vi "PCO_GetHWIOSignal.vi"(8 "error in (no error)":errorcluster {"code" format="%x"}, 10 "wSignalNum":u16, 11 "ph":u64) -> (0 "error out":errorcluster {"code" format="%x"}, 1 "strSignal":T1, 2 "ErrorMessage":i32 format="%x", 3 "ph out":u64)   [LabVIEW 2019, in "SDK.lvlib" / "TimingControl.lvlib"]
doc: "<b>Description:</b>\nThis function returns the current settings of a distinct hardware input/output (IO) signal line. To select the setting for a signal line use PCO_SetHWIOSignal.\n\n<b>Supported camera type:</b>\npco.edge, pco.dimax\n\n<b>Descriptor dependency:</b>\ndwGeneralCapsDESC1: HW_IO_SIGNAL_DESCRIPTOR"
uses:
  TimingControl.lvlib
  Structures/Structures.lvlib
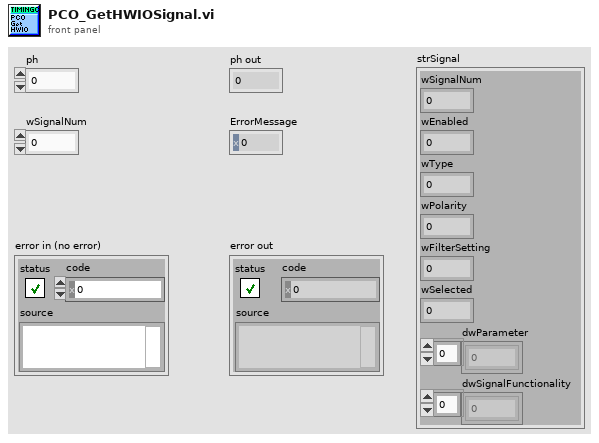
[diagram p1: front panel]
types:
  T1 = cluster{"wSignalNum":u16, "wEnabled":u16, "wType":u16, "wPolarity":u16, "wFilterSetting":u16, "wSelected":u16, "dwParameter":u32[], "dwSignalFunctionality":u32[]}
  T2 = cluster{"wSize":u16, "wSignalNum":u16, "wEnabled":u16, "wType":u16, "wPolarity":u16, "wFilterSetting":u16, "wSelected":u16, "ZZwReserved":u16, "dwParameter":cluster{u32, u32, u32, u32}, "dwSignalFunctionality":cluster{u32, u32, u32, u32}, "ZZdwReserved":cluster{u32, u32, u32}}
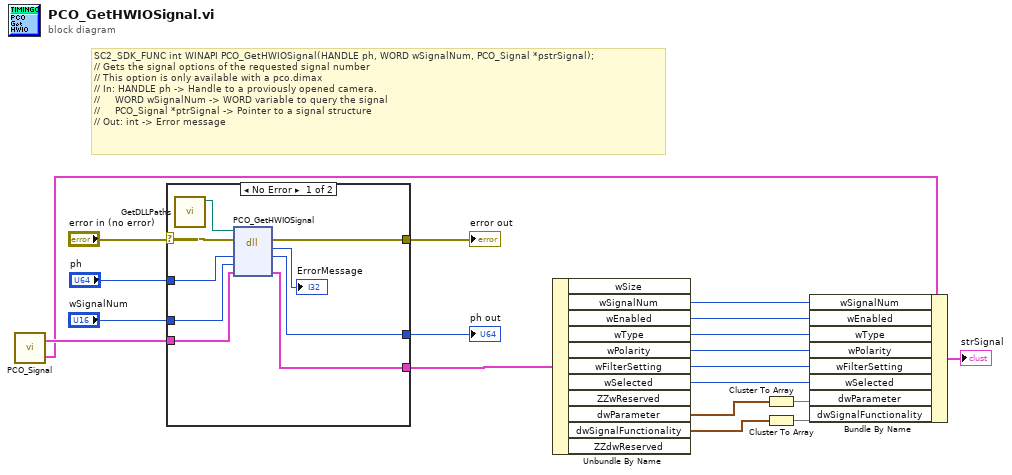
[diagram p0: block diagram]
diagram:
  # "SC2_SDK_FUNC int WINAPI PCO_GetHWIOSignal(HANDLE ph, WORD wSignalNum, PCO_Signal *pstrSignal);\n// Gets the signal options of the requested signal number\n// This option is only available with a pco.dimax\n// In: HANDLE ph -> Handle to a proviously opened camera.\n//     WORD wSignalNum -> WORD variable to query the signal\n//     PCO_Signal *ptrSignal -> Pointer to a signal structure\n// Out: int -> Error message"
  n1 = call "PCO_Signal.vi"() -> ("PCO_Signal"=w12:T1, "PCO_Signal_Raw"=w15:T2)  [unwired: 4 in, 2 out]
  n2 = case shown="No Error" "error in (no error)" {
    selector: "error in (no error)" -> [w22 w31]
    tunnel: "ph" -> [w27 w30]
    tunnel: [w26 w30] -> w18
    tunnel: "wSignalNum" -> [w25 _]
    tunnel: [w24 w31] -> w16
    tunnel: w15 -> [w23 w29]
    tunnel: [w21 w29] -> w13
    frame No Error {
      n3 = call "GetDLLPaths.vi"() -> ("SC2_Cam_Path"=w20:path)  [unwired: 8 in, 3 out]
      n4 = dll-call lib="?" fn="PCO_GetHWIOSignal"(path in=w20, error in=w22, "ph"=w27, "wSignalNum"=w25, "pstrSignal"=w23) -> (error out=w24:errorcluster, "return type"=→"ErrorMessage":i32, "ph"=w26:u64, "pstrSignal"=w21:T2)  [unwired: 2 in, 1 out]
    }
    frame Error {
    }
  }
  "ph out" <- w18
  "error out" <- w16
  n5 = Unbundle By Name(w13) -> ("wSignalNum"=w11:u16, "wEnabled"=w10:u16, "wType"=w9:u16, "wPolarity"=w8:u16, "wFilterSetting"=w7:u16, "wSelected"=w6:u16, "dwParameter"=w5:cluster{u32, u32, u32, u32}, "dwSignalFunctionality"=w3:cluster{u32, u32, u32, u32})  [unwired: 3 out]
  n6 = Cluster To Array(cluster=w5) -> (array=w4:u32[])
  n7 = Cluster To Array(cluster=w3) -> (array=w2:u32[])
  n8 = Bundle By Name(cluster=w12, "wSignalNum"=w11, "wEnabled"=w10, "wType"=w9, "wPolarity"=w8, "wFilterSetting"=w7, "wSelected"=w6, "dwParameter"=w4, "dwSignalFunctionality"=w2) -> (→"strSignal":T1)
